vi "Read Step Analyze.vi"(11 "Data":string) -> (3 "AC Advance Step Data":T1 {"Transient Time" format="%.1f ms"; "Transient Site" format="%.0f ¢X"; "Transient Volt" format="%.1f V"; "CF Lo Limit" format="%.2f"; "CF Hi Limit" format="%.2f"; "Q Lo Limit" format="%.0f VAR"; "Q Hi Limit" format="%.0f VAR"; "VA Lo Limit" format="%.0f VA"; "VA Hi Limit" format="%.0f VA"; "PF Lo Limit" format="%.3f"; "PF Hi Limit" format="%.3f"; "P Lo Limit" format="%.0f W"; "P Hi Limit" format="%.0f W"; "AP Lo Limit" format="%.1f A"; "AP Hi Limit" format="%.1f A"; "A Lo Limit" format="%.2f A"; "A Hi Limit" format="%.2f A"; "Delay Time" format="%.1f s"; "£GT" format="%.0f ms"; "£GF" format="%.1f Hz"; "£GV" format="%.1f V"; "Time" format="%.1f s"; "Voltage" format="%.1f V"; "Frequency" format="%.1f Hz"})   [LabVIEW 2013]
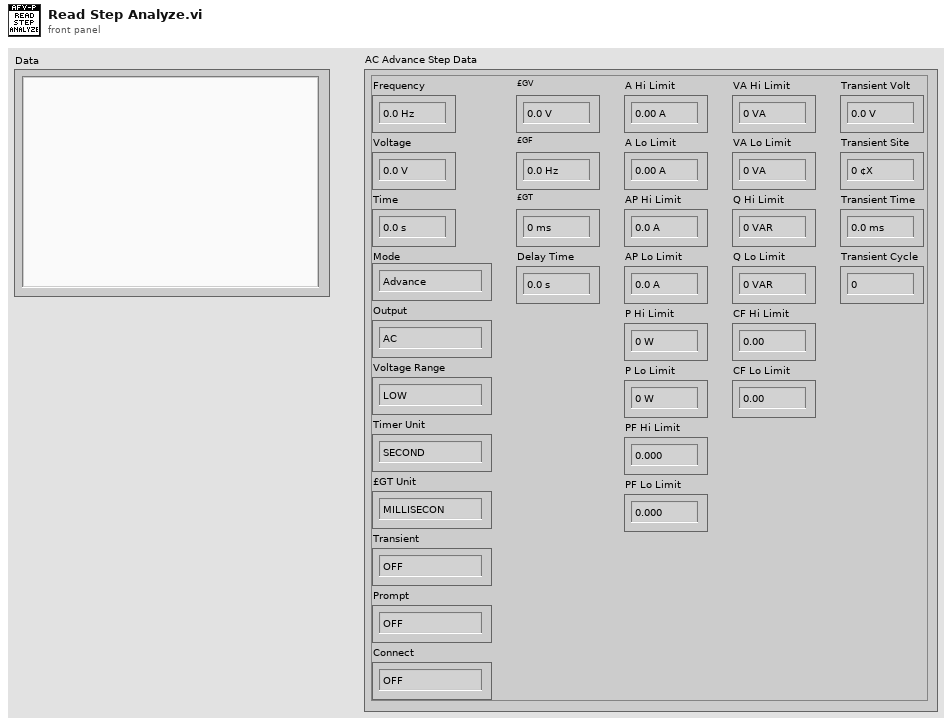
[diagram p1: front panel]
types:
  T1 = cluster{"Frequency":dbl, "Voltage":dbl, "Time":dbl, "Mode":enum16{"Advance", "Basic"}, "Output":enum16{"AC", "DC"}, "Voltage Range":enum16{"LOW", "HIGH", "AUTO"}, "Timer Unit":enum16{"SECOND", "MINUTE", "HOUR"}, "£GT Unit":enum16{"MILLISECON", "SECOND", "CYCLE"}, "Transient":enum16{"OFF", "ON"}, "Prompt":enum16{"OFF", "ON"}, "Connect":enum16{"OFF", "ON"}, "£GV":dbl, "£GF":dbl, "£GT":u16, "Delay Time":dbl, "A Hi Limit":dbl, "A Lo Limit":dbl, "AP Hi Limit":dbl, "AP Lo Limit":dbl, "P Hi Limit":u16, "P Lo Limit":u16, "PF Hi Limit":dbl, "PF Lo Limit":dbl, "VA Hi Limit":u16, "VA Lo Limit":u16, "Q Hi Limit":u16, "Q Lo Limit":u16, "CF Hi Limit":dbl, "CF Lo Limit":dbl, "Transient Volt":dbl, "Transient Site":u16, "Transient Time":dbl, "Transient Cycle":u16}
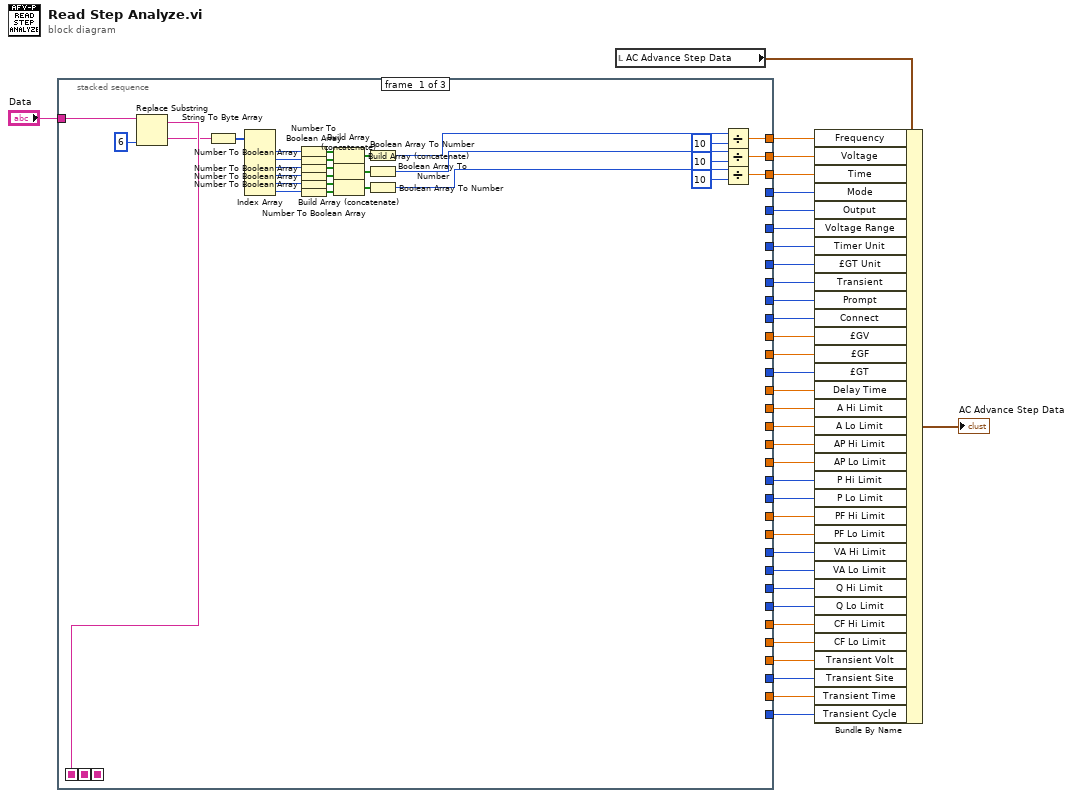
[diagram p0: block diagram]
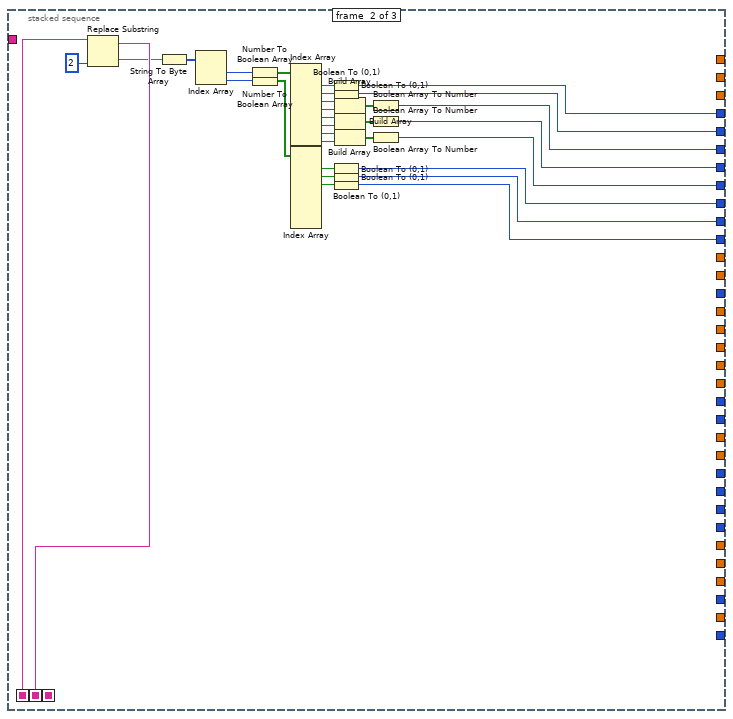
[diagram p2: hidden frame]
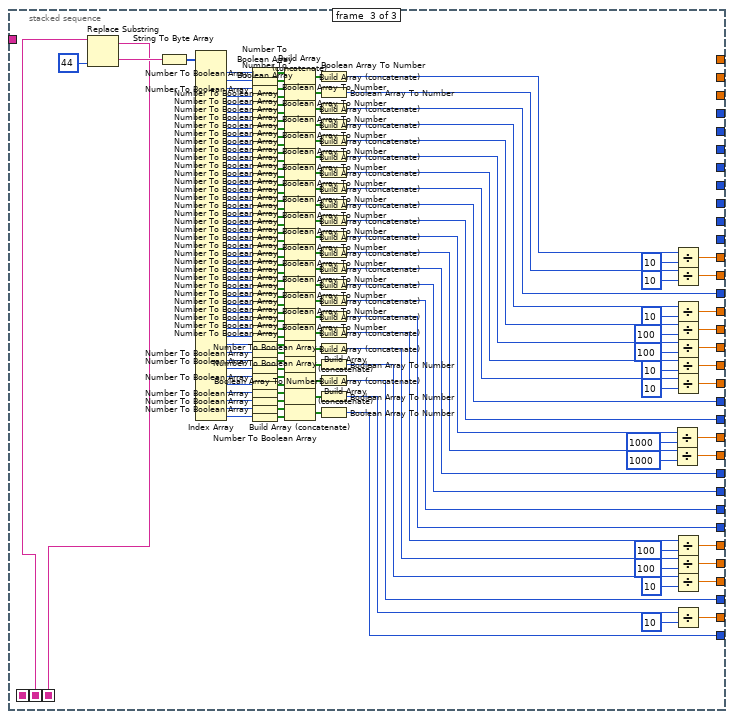
[diagram p3: hidden frame]
diagram:
  n1 = stacked-sequence {
    seq-local: [w64 _ _] -> [_ w94 _]
    seq-local: [_ w95 _] -> [_ _ w240]
    seq-local: [_ _ w241] -> [_ _ _]
    tunnel: [w42 _ _] -> w35
    tunnel: [w41 _ _] -> w34
    tunnel: [w38 _ _] -> w33
    tunnel: [_ w78 _] -> w32
    tunnel: [_ w77 _] -> w31
    tunnel: [_ w76 _] -> w30
    tunnel: [_ w75 _] -> w29
    tunnel: [_ w74 _] -> w28
    tunnel: [_ w73 _] -> w27
    tunnel: [_ w72 _] -> w26
    tunnel: [_ w71 _] -> w25
    tunnel: [_ _ w135] -> w24
    tunnel: [_ _ w131] -> w23
    tunnel: [_ _ w239] -> w22
    tunnel: [_ _ w129] -> w21
    tunnel: [_ _ w125] -> w20
    tunnel: [_ _ w123] -> w19
    tunnel: [_ _ w120] -> w18
    tunnel: [_ _ w118] -> w17
    tunnel: [_ _ w173] -> w16
    tunnel: [_ _ w142] -> w15
    tunnel: [_ _ w113] -> w14
    tunnel: [_ _ w112] -> w13
    tunnel: [_ _ w141] -> w12
    tunnel: [_ _ w140] -> w11
    tunnel: [_ _ w139] -> w10
    tunnel: [_ _ w107] -> w9
    tunnel: [_ _ w104] -> w8
    tunnel: [_ _ w103] -> w7
    tunnel: [_ _ w99] -> w6
    tunnel: [_ _ w138] -> w5
    tunnel: [_ _ w97] -> w4
    tunnel: [_ _ w137] -> w3
    tunnel: "Data" -> [w46 _ _]
    frame #0 {
      n2 = Replace Substring(2:6 ("length (len. of substring)"), 5:w46) -> (0:w57:string, 1:w64:string)  [unwired: 2 in]
      n3 = String To Byte Array(string=w57) -> (unsigned byte array=w58:u8[])
      n4 = Index Array(array=w58) -> (element #1=w62:u8, element #2=w63:u8, element #3=w53:u8, element #4=w52:u8, element #5=w48:u8, element #6=w47:u8)  [unwired: 6 in]
      n5 = Number To Boolean Array(number=w62) -> (Boolean array=w60:bool[])
      n6 = Number To Boolean Array(number=w63) -> (Boolean array=w61:bool[])
      n7 = Number To Boolean Array(number=w53) -> (Boolean array=w55:bool[])
      n8 = Number To Boolean Array(number=w52) -> (Boolean array=w54:bool[])
      n9 = Number To Boolean Array(number=w48) -> (Boolean array=w50:bool[])
      n10 = Number To Boolean Array(number=w47) -> (Boolean array=w51:bool[])
      n11 = Build Array (concatenate)(w60, w61) -> (w59:bool[])
      n12 = Build Array (concatenate)(w55, w54) -> (w56:bool[])
      n13 = Build Array (concatenate)(w50, w51) -> (w49:bool[])
      n14 = Boolean Array To Number(Boolean array=w59) -> (number=w45:u32)
      n15 = Boolean Array To Number(Boolean array=w56) -> (number=w40:u32)
      n16 = Boolean Array To Number(Boolean array=w49) -> (number=w37:u32)
      n17 = Divide(x=w45, y=u32 10) -> (x/y=w42:dbl)
      n18 = Divide(x=w40, y=u32 10) -> (x/y=w41:dbl)
      n19 = Divide(x=w37, y=u32 10) -> (x/y=w38:dbl)
    }
    frame #1 {
      n20 = Replace Substring(2:2 ("length (len. of substring)"), 5:w94) -> (0:w90:string, 1:w95:string)  [unwired: 2 in]
      n21 = String To Byte Array(string=w90) -> (unsigned byte array=w92:u8[])
      n22 = Index Array(array=w92) -> (element #1=w91:u8, element #2=w70:u8)  [unwired: 2 in]
      n23 = Number To Boolean Array(number=w91) -> (Boolean array=w93:bool[])
      n24 = Number To Boolean Array(number=w70) -> (Boolean array=w69:bool[])
      n25 = Index Array(array=w93) -> (element #1=w89:bool, element #2=w88:bool, element #3=w86:bool, element #4=w85:bool, element #5=w83:bool, element #6=w82:bool, element #7=w80:bool, element #8=w79:bool)  [unwired: 8 in]
      n26 = Index Array(array=w69) -> (element #1=w68:bool, element #2=w67:bool, element #3=w66:bool)  [unwired: 8 in, 5 out]
      n27 = Boolean To (0,1)(Boolean=w89) -> (0, 1=w78:i16)
      n28 = Boolean To (0,1)(Boolean=w88) -> (0, 1=w77:i16)
      n29 = Boolean To (0,1)(Boolean=w68) -> (0, 1=w73:i16)
      n30 = Boolean To (0,1)(Boolean=w67) -> (0, 1=w72:i16)
      n31 = Boolean To (0,1)(Boolean=w66) -> (0, 1=w71:i16)
      n32 = Build Array(w86, w85) -> (w87:bool[])
      n33 = Build Array(w83, w82) -> (w84:bool[])
      n34 = Build Array(w80, w79) -> (w81:bool[])
      n35 = Boolean Array To Number(Boolean array=w87) -> (number=w76:u32)
      n36 = Boolean Array To Number(Boolean array=w84) -> (number=w75:u32)
      n37 = Boolean Array To Number(Boolean array=w81) -> (number=w74:u32)
    }
    frame #2 {
      n38 = Replace Substring(2:44 ("length (len. of substring)"), 5:w240) -> (0:w252:string, 1:w241:string)  [unwired: 2 in]
      n39 = String To Byte Array(string=w252) -> (unsigned byte array=w253:u8[])
      n40 = Index Array(array=w253) -> (element #1=w257:u8, element #2=w258:u8, element #3=w248:u8, element #4=w247:u8, element #5=w243:u8, element #6=w242:u8, element #7=w235:u8, element #8=w234:u8, element #9=w221:u8, element #10=w220:u8, element #11=w219:u8, element #12=w218:u8, element #13=w217:u8, element #14=w216:u8, element #15=w215:u8, element #16=w214:u8, element #17=w189:u8, element #18=w188:u8, element #19=w187:u8, element #20=w186:u8, element #21=w185:u8, element #22=w184:u8, element #23=w183:u8, element #24=w182:u8, element #25=w181:u8, element #26=w180:u8, element #27=w179:u8, element #28=w178:u8, element #29=w177:u8, element #30=w176:u8, element #31=w175:u8, element #32=w174:u8, element #33=w163:u8, element #34=w162:u8, element #35=w161:u8, element #36=w160:u8, element #37=w159:u8, element #38=w158:u8, element #39=w148:u8, element #40=w147:u8, element #41=w146:u8, element #42=w145:u8, element #43=w144:u8, element #44=w143:u8)  [unwired: 44 in]
      n41 = Number To Boolean Array(number=w257) -> (Boolean array=w255:bool[])
      n42 = Number To Boolean Array(number=w258) -> (Boolean array=w256:bool[])
      n43 = Number To Boolean Array(number=w248) -> (Boolean array=w250:bool[])
      n44 = Number To Boolean Array(number=w247) -> (Boolean array=w249:bool[])
      n45 = Number To Boolean Array(number=w243) -> (Boolean array=w245:bool[])
      n46 = Number To Boolean Array(number=w242) -> (Boolean array=w246:bool[])
      n47 = Number To Boolean Array(number=w235) -> (Boolean array=w237:bool[])
      n48 = Number To Boolean Array(number=w234) -> (Boolean array=w236:bool[])
      n49 = Number To Boolean Array(number=w221) -> (Boolean array=w223:bool[])
      n50 = Number To Boolean Array(number=w220) -> (Boolean array=w222:bool[])
      n51 = Number To Boolean Array(number=w219) -> (Boolean array=w226:bool[])
      n52 = Number To Boolean Array(number=w218) -> (Boolean array=w227:bool[])
      n53 = Number To Boolean Array(number=w217) -> (Boolean array=w229:bool[])
      n54 = Number To Boolean Array(number=w216) -> (Boolean array=w228:bool[])
      n55 = Number To Boolean Array(number=w215) -> (Boolean array=w232:bool[])
      n56 = Number To Boolean Array(number=w214) -> (Boolean array=w233:bool[])
      n57 = Number To Boolean Array(number=w189) -> (Boolean array=w191:bool[])
      n58 = Number To Boolean Array(number=w188) -> (Boolean array=w190:bool[])
      n59 = Number To Boolean Array(number=w187) -> (Boolean array=w194:bool[])
      n60 = Number To Boolean Array(number=w186) -> (Boolean array=w195:bool[])
      n61 = Number To Boolean Array(number=w185) -> (Boolean array=w197:bool[])
      n62 = Number To Boolean Array(number=w184) -> (Boolean array=w196:bool[])
      n63 = Number To Boolean Array(number=w183) -> (Boolean array=w200:bool[])
      n64 = Number To Boolean Array(number=w182) -> (Boolean array=w201:bool[])
      n65 = Number To Boolean Array(number=w181) -> (Boolean array=w212:bool[])
      n66 = Number To Boolean Array(number=w180) -> (Boolean array=w213:bool[])
      n67 = Number To Boolean Array(number=w179) -> (Boolean array=w209:bool[])
      n68 = Number To Boolean Array(number=w178) -> (Boolean array=w208:bool[])
      n69 = Number To Boolean Array(number=w177) -> (Boolean array=w206:bool[])
      n70 = Number To Boolean Array(number=w176) -> (Boolean array=w207:bool[])
      n71 = Number To Boolean Array(number=w175) -> (Boolean array=w203:bool[])
      n72 = Number To Boolean Array(number=w174) -> (Boolean array=w202:bool[])
      n73 = Number To Boolean Array(number=w163) -> (Boolean array=w165:bool[])
      n74 = Number To Boolean Array(number=w162) -> (Boolean array=w166:bool[])
      n75 = Number To Boolean Array(number=w161) -> (Boolean array=w168:bool[])
      n76 = Number To Boolean Array(number=w160) -> (Boolean array=w167:bool[])
      n77 = Number To Boolean Array(number=w159) -> (Boolean array=w171:bool[])
      n78 = Number To Boolean Array(number=w158) -> (Boolean array=w172:bool[])
      n79 = Number To Boolean Array(number=w148) -> (Boolean array=w150:bool[])
      n80 = Number To Boolean Array(number=w147) -> (Boolean array=w151:bool[])
      n81 = Number To Boolean Array(number=w146) -> (Boolean array=w156:bool[])
      n82 = Number To Boolean Array(number=w145) -> (Boolean array=w155:bool[])
      n83 = Number To Boolean Array(number=w144) -> (Boolean array=w153:bool[])
      n84 = Number To Boolean Array(number=w143) -> (Boolean array=w154:bool[])
      n85 = Build Array (concatenate)(w255, w256) -> (w254:bool[])
      n86 = Build Array (concatenate)(w250, w249) -> (w251:bool[])
      n87 = Build Array (concatenate)(w245, w246) -> (w244:bool[])
      n88 = Build Array (concatenate)(w237, w236) -> (w238:bool[])
      n89 = Build Array (concatenate)(w223, w222) -> (w224:bool[])
      n90 = Build Array (concatenate)(w226, w227) -> (w225:bool[])
      n91 = Build Array (concatenate)(w229, w228) -> (w230:bool[])
      n92 = Build Array (concatenate)(w232, w233) -> (w231:bool[])
      n93 = Build Array (concatenate)(w191, w190) -> (w192:bool[])
      n94 = Build Array (concatenate)(w194, w195) -> (w193:bool[])
      n95 = Build Array (concatenate)(w197, w196) -> (w198:bool[])
      n96 = Build Array (concatenate)(w200, w201) -> (w199:bool[])
      n97 = Build Array (concatenate)(w212, w213) -> (w211:bool[])
      n98 = Build Array (concatenate)(w209, w208) -> (w210:bool[])
      n99 = Build Array (concatenate)(w206, w207) -> (w205:bool[])
      n100 = Build Array (concatenate)(w203, w202) -> (w204:bool[])
      n101 = Build Array (concatenate)(w165, w166) -> (w164:bool[])
      n102 = Build Array (concatenate)(w168, w167) -> (w169:bool[])
      n103 = Build Array (concatenate)(w171, w172) -> (w170:bool[])
      n104 = Build Array (concatenate)(w150, w151) -> (w149:bool[])
      n105 = Build Array (concatenate)(w156, w155) -> (w157:bool[])
      n106 = Build Array (concatenate)(w153, w154) -> (w152:bool[])
      n107 = Boolean Array To Number(Boolean array=w254) -> (number=w136:u32)
      n108 = Boolean Array To Number(Boolean array=w251) -> (number=w132:u32)
      n109 = Boolean Array To Number(Boolean array=w244) -> (number=w239:u32)
      n110 = Boolean Array To Number(Boolean array=w238) -> (number=w130:u32)
      n111 = Boolean Array To Number(Boolean array=w224) -> (number=w126:u32)
      n112 = Boolean Array To Number(Boolean array=w225) -> (number=w122:u32)
      n113 = Boolean Array To Number(Boolean array=w230) -> (number=w119:u32)
      n114 = Boolean Array To Number(Boolean array=w231) -> (number=w117:u32)
      n115 = Boolean Array To Number(Boolean array=w192) -> (number=w173:u32)
      n116 = Boolean Array To Number(Boolean array=w193) -> (number=w142:u32)
      n117 = Boolean Array To Number(Boolean array=w198) -> (number=w114:u32)
      n118 = Boolean Array To Number(Boolean array=w199) -> (number=w111:u32)
      n119 = Boolean Array To Number(Boolean array=w211) -> (number=w141:u32)
      n120 = Boolean Array To Number(Boolean array=w210) -> (number=w140:u32)
      n121 = Boolean Array To Number(Boolean array=w205) -> (number=w139:u32)
      n122 = Boolean Array To Number(Boolean array=w204) -> (number=w107:u32)
      n123 = Boolean Array To Number(Boolean array=w164) -> (number=w105:u32)
      n124 = Boolean Array To Number(Boolean array=w169) -> (number=w106:u32)
      n125 = Boolean Array To Number(Boolean array=w170) -> (number=w100:u32)
      n126 = Boolean Array To Number(Boolean array=w149) -> (number=w138:u32)
      n127 = Boolean Array To Number(Boolean array=w157) -> (number=w98:u32)
      n128 = Boolean Array To Number(Boolean array=w152) -> (number=w137:u32)
      n129 = Divide(x=w114, y=u32 1000) -> (x/y=w113:dbl)
      n130 = Divide(x=w111, y=u32 1000) -> (x/y=w112:dbl)
      n131 = Divide(x=w136, y=u32 10) -> (x/y=w135:dbl)
      n132 = Divide(x=w132, y=u32 10) -> (x/y=w131:dbl)
      n133 = Divide(x=w130, y=u32 10) -> (x/y=w129:dbl)
      n134 = Divide(x=w126, y=u32 100) -> (x/y=w125:dbl)
      n135 = Divide(x=w122, y=u32 100) -> (x/y=w123:dbl)
      n136 = Divide(x=w119, y=u32 10) -> (x/y=w120:dbl)
      n137 = Divide(x=w117, y=u32 10) -> (x/y=w118:dbl)
      n138 = Divide(x=w105, y=u32 100) -> (x/y=w104:dbl)
      n139 = Divide(x=w106, y=u32 100) -> (x/y=w103:dbl)
      n140 = Divide(x=w100, y=u32 10) -> (x/y=w99:dbl)
      n141 = Divide(x=w98, y=u32 10) -> (x/y=w97:dbl)
    }
  }
  n142 = local read "AC Advance Step Data"() -> (w36:T1)
  n143 = Bundle By Name(cluster=w36, "Frequency"=w35, "Voltage"=w34, "Time"=w33, "Mode"=w32, "Output"=w31, "Voltage Range"=w30, "Timer Unit"=w29, "£GT Unit"=w28, "Transient"=w27, "Prompt"=w26, "Connect"=w25, "£GV"=w24, "£GF"=w23, "£GT"=w22, "Delay Time"=w21, "A Hi Limit"=w20, "A Lo Limit"=w19, "AP Hi Limit"=w18, "AP Lo Limit"=w17, "P Hi Limit"=w16, "P Lo Limit"=w15, "PF Hi Limit"=w14, "PF Lo Limit"=w13, "VA Hi Limit"=w12, "VA Lo Limit"=w11, "Q Hi Limit"=w10, "Q Lo Limit"=w9, "CF Hi Limit"=w8, "CF Lo Limit"=w7, "Transient Volt"=w6, "Transient Site"=w5, "Transient Time"=w4, "Transient Cycle"=w3) -> (→"AC Advance Step Data":T1)
